vi "WriteRegHack.vi"() -> ()   [LabVIEW 2020]
uses:
  <vilib>/Plasmionique/MB Master/MB_PDU/MB_PDU_Cluster.ctl
  <vilib>/Plasmionique/MB Master/MB_Master_TCP/MB_Master_TCP.lvclass
  <vilib>/Plasmionique/MB Master/MB Master.lvlib
panel:
  in  "autoPacket":bool
  in  "MB_PDU":T1={"Function Code"=1, "Data"=[], "RTU_DataBytes"=0} {"Data" format="%02x"; "Function Code" format="%.0x"}
  in  "values":u16[](array[numeric])
  in  "starting address":u16
  out "error out 2":errorcluster
  in  "IP Address(:port)":string
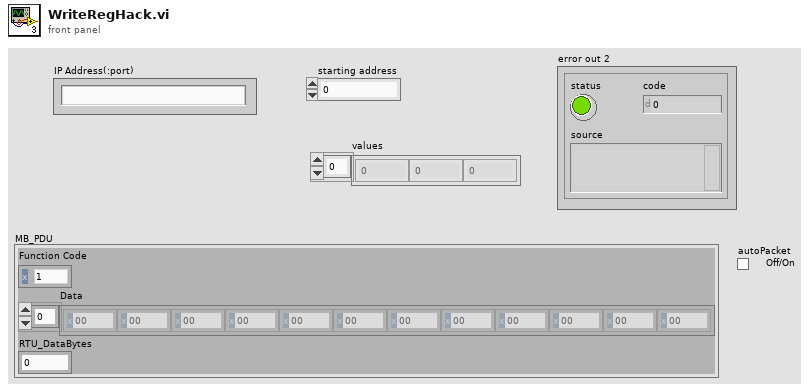
[diagram p1: front panel]
types:
  T1 = typedef "MB Master.lvlib/MB_PDU_Cluster.ctl" = cluster{"Function Code":u8, "Data":u8[], "RTU_DataBytes":i32}
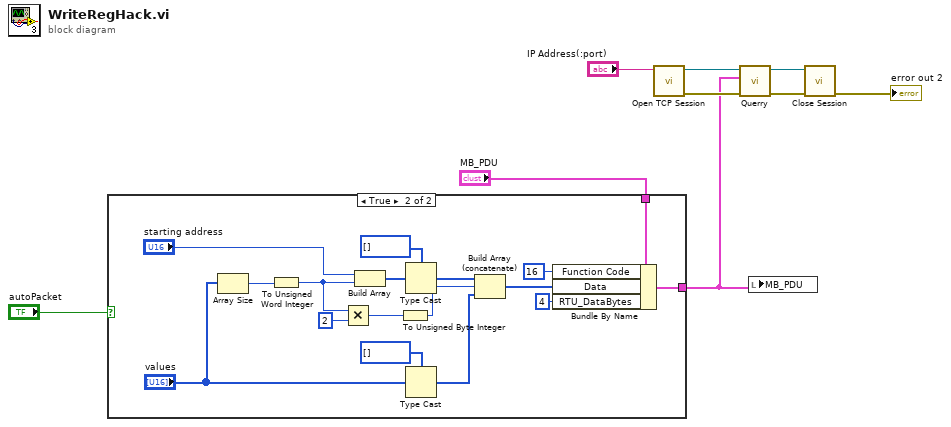
[diagram p0: block diagram]
diagram:
  n1 = case shown="True" "autoPacket" {
    tunnel: [w10 w27] -> w1
    tunnel: "MB_PDU" -> [w10 w26]
    frame False {
    }
    frame True {
      n2 = Array Size(array="values") -> (size(s)=w13:i32)
      n3 = To Unsigned Word Integer(number=w13) -> (unsigned 16bit integer=w12:u16)
      n4 = Multiply(x=w12, y=u16 2) -> (x*y=w20:u16)
      n5 = Build Array("starting address", w12) -> (w25:u16[])
      n6 = To Unsigned Byte Integer(number=w20) -> (unsigned 8bit integer=w18:u8)
      n7 = Type Cast(type=u8[] [], x=w25) -> (*(type *) &x=w19:u8[])
      n8 = Type Cast(type=u8[] [], x="values") -> (*(type *) &x=w16:u8[])
      n9 = Build Array (concatenate)(w19, w18, w16) -> (w15:u8[])
      n10 = Bundle By Name(cluster=w26, "Function Code"=u8 16, "Data"=w15, "RTU_DataBytes"=4 ("NumBytes")) -> (w27:T1)
    }
  }
  n11 = call <vilib>:"Open TCP Session.vi"("IP Address"="IP Address(:port)") -> ("error out"=w4:errorcluster, "MB_TCP session"=w8:refnum<class "MB_Master_TCP.lvclass">)  [unwired: 9 in]
  n12 = call-dynamic "Querry.vi"("error in (no error)"=w4, "PDU_req"=w1, "MB_Master_TCP in"=w8) -> ("error out"=w6:errorcluster, "MB_Master_TCP out"=w7:refnum<class "MB_Master_TCP.lvclass">)  [unwired: 6 in, 1 out]
  n13 = local write "MB_PDU"(w1) -> ()
  n14 = call-dynamic "Close Session.vi"("error in (no error)"=w6, "MB TCP session"=w7) -> ("error out"=→"error out 2":errorcluster)  [unwired: 9 in]
